vi "setVerticalChannelToHW.vi"(8 "error in (no error)":errorcluster, 11 "TektronixDPO in":refnum<class "TektronixDPO.lvclass">) -> (0 "error out":errorcluster, 3 "TektronixDPO out":refnum<class "TektronixDPO.lvclass">)   [LabVIEW 2013, in "TektronixDPO.lvclass"]
doc: "Send the channel settings to the physical device and read them back from it"
uses:
  TektronixDPO.lvclass
  TektronixDPO.lvclass/TektronixDPO.ctl
  SupportClasses/TektronixDPOPhysicalDevice/TektronixDPO_PhysicalDevice.lvclass
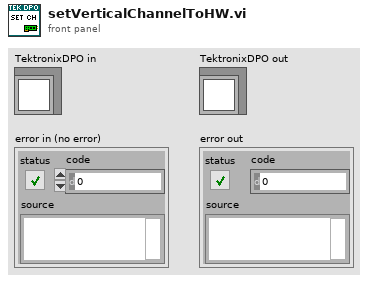
[diagram p1: front panel]
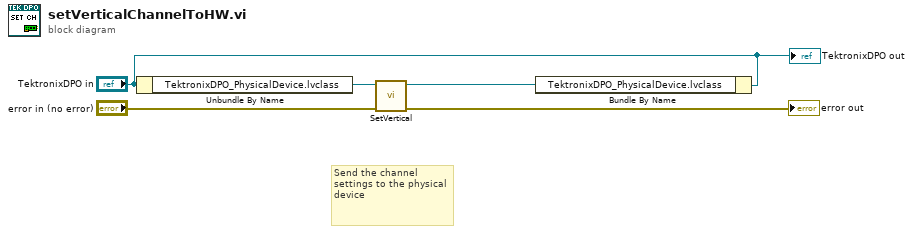
[diagram p0: block diagram]
diagram:
  # "Send the channel settings to the physical device"
  n1 = Unbundle By Name("TektronixDPO in") -> ("TektronixDPO_PhysicalDevice.lvclass"=w4:refnum<class "TektronixDPO_PhysicalDevice.lvclass">)
  n2 = call "SetVertical.vi"("error in (no error)"="error in (no error)", "TektronixDPO in"=w4) -> ("error out"=→"error out":errorcluster, "TektronixDPO_PhysicalDevice.lvclass"=w1:refnum<class "TektronixDPO_PhysicalDevice.lvclass">)  [unwired: 8 in]
  n3 = Bundle By Name(cluster="TektronixDPO in", "TektronixDPO_PhysicalDevice.lvclass"=w1) -> ()  [unwired: 1 out]
  "TektronixDPO out" <- "TektronixDPO in"
